vi "HFRR ADV v07 new software.vi"() -> ()   [LabVIEW 2025] (continued)
              n1803 = String Subset(string=w2037, offset (0)=85) -> (substring=w2039:string)  [unwired: 1 in]
              n1804 = String Subset(string=w2037, offset (0)=35, length (rest)=9 ("length (rest)")) -> (substring=w2060:string)
              n1805 = String Subset(string=w2037, offset (0)=55, length (rest)=9 ("length (rest)")) -> (substring=w2045:string)
              n1806 = String Subset(string=w2037, offset (0)=25) -> (substring=w2041:string)  [unwired: 1 in]
              n1807 = String Subset(string=w2037, offset (0)=15, length (rest)=9 ("length (rest)")) -> (substring=w2066:string)
              n1808 = String Subset(string=w2037, offset (0)=0, length (rest)=14 ("length (rest)")) -> (substring=w2063:string)
              n1809 = String Subset(string=w2037, offset (0)=45, length (rest)=9 ("length (rest)")) -> (substring=w2050:string)
              n1810 = String Subset(string=w2037, offset (0)=65, length (rest)=9 ("length (rest)")) -> (substring=w2056:string)
              n1811 = Fract/Exp String To Number(string=w2039) -> (number=w2036:dbl)  [unwired: 3 in, 1 out]
              n1812 = Fract/Exp String To Number(string=w2060) -> (number=w2058:dbl)  [unwired: 3 in, 1 out]
              n1813 = Fract/Exp String To Number(string=w2045) -> (number=w2043:dbl)  [unwired: 3 in, 1 out]
              n1814 = Fract/Exp String To Number(string=w2041) -> (number=w2040:dbl)  [unwired: 3 in, 1 out]
              n1815 = Fract/Exp String To Number(string=w2066) -> (number=w2057:dbl)  [unwired: 3 in, 1 out]
              n1816 = Fract/Exp String To Number(string=w2063) -> (number=w2059:dbl)  [unwired: 3 in, 1 out]
              n1817 = Fract/Exp String To Number(string=w2050) -> (number=w2047:dbl)  [unwired: 3 in, 1 out]
              n1818 = Fract/Exp String To Number(string=w2056) -> (number=w2053:dbl)  [unwired: 3 in, 1 out]
              n1819 = Add(x=w2053, y=0.0) -> (x+y=w2051:dbl)
            }
            n1820 = String To Path(string=w1896) -> (path=w1994:path)
            n1821 = String To Path(string=w1894) -> (path=w1988:path)
            n1822 = local read "Numeric 11"() -> (w1978:i32)
            n1823 = local read "Numeric 13"() -> (w1980:i32)
            n1824 = Open/Create/Replace File "Open File"(file path (use dialog)=w1994) -> (refnum out=w1992:refnum<file>, error out=w1991:errorcluster)  [unwired: 5 in, 1 out]
            n1825 = Open/Create/Replace File "Open File"(file path (use dialog)=w1988) -> (refnum out=w1987:refnum<file>, error out=w1986:errorcluster)  [unwired: 5 in, 1 out]
            n1826 = for {
              N: w1978 -> [_]
              tunnel: w1992 -> [w2107]
              tunnel: w1991 -> [w2106]
              tunnel: [w2096] -> w1958 mode=indexing
              tunnel: [w2094] -> w1956 mode=indexing
              tunnel: [w2095] -> w1951 mode=indexing
              tunnel: w1977 -> [_]
              tunnel: [w2088] -> w1953 mode=indexing
              tunnel: [w2084] -> w1929 mode=indexing
              tunnel: [w2080] -> w1904 mode=indexing
              tunnel: [w2076] -> w1885 mode=indexing
              tunnel: [w2071] -> w1843 mode=indexing
              (unwired) TRUE ("line mode (F)")
              n1827 = Read from Text File "Read File"(file (use dialog)=w2107, error in=w2106) -> (text=w2072:string)  [unwired: 2 in, 3 out]
              n1828 = local write "String 7"(w2072) -> ()
              n1829 = String Subset(string=w2072, offset (0)=85, length (rest)=9 ("length (rest)")) -> (substring=w2075:string)
              n1830 = String Subset(string=w2072, offset (0)=35, length (rest)=9 ("length (rest)")) -> (substring=w2097:string)
              n1831 = String Subset(string=w2072, offset (0)=55, length (rest)=9 ("length (rest)")) -> (substring=w2083:string)
              n1832 = String Subset(string=w2072, offset (0)=25, length (rest)=9 ("length (rest)")) -> (substring=w2077:string)
              n1833 = String Subset(string=w2072, offset (0)=45, length (rest)=9 ("length (rest)")) -> (substring=w2085:string)
              n1834 = String Subset(string=w2072, offset (0)=0, length (rest)=14 ("length (rest)")) -> (substring=w2100:string)
              n1835 = String Subset(string=w2072, offset (0)=15, length (rest)=9 ("length (rest)")) -> (substring=w2103:string)
              n1836 = String Subset(string=w2072, offset (0)=65, length (rest)=9 ("length (rest)")) -> (substring=w2089:string)
              n1837 = Fract/Exp String To Number(string=w2075) -> (number=w2071:dbl)  [unwired: 3 in, 1 out]
              n1838 = Fract/Exp String To Number(string=w2097) -> (number=w2095:dbl)  [unwired: 3 in, 1 out]
              n1839 = Fract/Exp String To Number(string=w2083) -> (number=w2080:dbl)  [unwired: 3 in, 1 out]
              n1840 = Fract/Exp String To Number(string=w2077) -> (number=w2076:dbl)  [unwired: 3 in, 1 out]
              n1841 = Fract/Exp String To Number(string=w2085) -> (number=w2084:dbl)  [unwired: 3 in, 1 out]
              n1842 = Fract/Exp String To Number(string=w2100) -> (number=w2096:dbl)  [unwired: 3 in, 1 out]
              n1843 = Fract/Exp String To Number(string=w2103) -> (number=w2094:dbl)  [unwired: 3 in, 1 out]
              n1844 = Fract/Exp String To Number(string=w2089) -> (number=w2092:dbl)  [unwired: 3 in, 1 out]
              n1845 = Add(x=w2092, y=0.0) -> (x+y=w2088:dbl)
            }
            n1846 = for {
              N: w1980 -> [_]
              tunnel: w1987 -> [w2035]
              tunnel: w1986 -> [w2034]
              tunnel: [w2024] -> w1940 mode=indexing
              tunnel: [w2023] -> w1933 mode=indexing
              tunnel: w1977 -> [_]
              tunnel: [w2012] -> w1938 mode=indexing
              tunnel: [w2017] -> w1935 mode=indexing
              tunnel: [w2013] -> w1925 mode=indexing
              tunnel: [w2008] -> w1900 mode=indexing
              tunnel: [w2004] -> w1881 mode=indexing
              tunnel: [w1999] -> w1841 mode=indexing
              (unwired) 1.0 ("x")
              (unwired) TRUE ("line mode (F)")
              n1847 = Read from Text File "Read File"(file (use dialog)=w2035, error in=w2034) -> (text=w2000:string)  [unwired: 2 in, 3 out]
              n1848 = local write "String 12"(w2000) -> ()
              n1849 = String Subset(string=w2000, offset (0)=85, length (rest)=9 ("length (rest)")) -> (substring=w2002:string)
              n1850 = String Subset(string=w2000, offset (0)=35, length (rest)=9 ("length (rest)")) -> (substring=w2025:string)
              n1851 = String Subset(string=w2000, offset (0)=55, length (rest)=9 ("length (rest)")) -> (substring=w2010:string)
              n1852 = String Subset(string=w2000, offset (0)=25, length (rest)=9 ("length (rest)")) -> (substring=w2006:string)
              n1853 = String Subset(string=w2000, offset (0)=45, length (rest)=9 ("length (rest)")) -> (substring=w2015:string)
              n1854 = String Subset(string=w2000, offset (0)=15, length (rest)=9 ("length (rest)")) -> (substring=w2031:string)
              n1855 = String Subset(string=w2000, offset (0)=0, length (rest)=14 ("length (rest)")) -> (substring=w2028:string)
              n1856 = String Subset(string=w2000, offset (0)=65, length (rest)=9 ("length (rest)")) -> (substring=w2018:string)
              n1857 = Fract/Exp String To Number(string=w2002) -> (number=w1999:dbl)  [unwired: 3 in, 1 out]
              n1858 = Fract/Exp String To Number(string=w2025) -> (number=w2023:dbl)  [unwired: 3 in, 1 out]
              n1859 = Fract/Exp String To Number(string=w2010) -> (number=w2008:dbl)  [unwired: 3 in, 1 out]
              n1860 = Fract/Exp String To Number(string=w2006) -> (number=w2004:dbl)  [unwired: 3 in, 1 out]
              n1861 = Fract/Exp String To Number(string=w2015) -> (number=w2013:dbl)  [unwired: 3 in, 1 out]
              n1862 = Fract/Exp String To Number(string=w2031) -> (number=w2012:dbl)  [unwired: 3 in, 1 out]
              n1863 = Fract/Exp String To Number(string=w2028) -> (number=w2024:dbl)  [unwired: 3 in, 1 out]
              n1864 = Fract/Exp String To Number(string=w2018) -> (number=w2021:dbl)  [unwired: 3 in, 1 out]
              n1865 = Add(x=w2021, y=0.0) -> (x+y=w2017:dbl)
            }
            n1866 = Delete From Array(array=w1883, index=0) -> (array with subset deleted=w1856:dbl[])  [unwired: 1 in, 1 out]
            n1867 = Delete From Array(array=w1946, index=0) -> (array with subset deleted=w1919:dbl[])  [unwired: 1 in, 1 out]
            n1868 = Delete From Array(array=w1926, index=0) -> (array with subset deleted=w1914:dbl[])  [unwired: 1 in, 1 out]
            n1869 = Delete From Array(array=w1944, index=0) -> (array with subset deleted=w1945:dbl[])  [unwired: 1 in, 1 out]
            n1870 = call-poly <vilib>:"Mean.vi"("X"=w1856) -> ("mean"=→"КОФ2 4":dbl)  [unwired: 1 out]
            n1871 = call-poly <vilib>:"Mean.vi"("X"=w1919) -> ("mean"=→"КОФ3":dbl)  [unwired: 1 out]
            n1872 = call-poly <vilib>:"Mean.vi"("X"=w1914) -> ("mean"=→"CP3":dbl)  [unwired: 1 out]
            n1873 = Delete From Array(array=w1908, index=0) -> (array with subset deleted=w1835:dbl[])  [unwired: 1 in, 1 out]
            n1874 = Delete From Array(array=w1847, index=0) -> (array with subset deleted=w1834:dbl[])  [unwired: 1 in, 1 out]
            n1875 = Delete From Array(array=w1887, index=0) -> (array with subset deleted=w1858:dbl[])  [unwired: 1 in, 1 out]
            n1876 = Delete From Array(array=w1965, index=0) -> (array with subset deleted=w1920:dbl[])  [unwired: 1 in, 1 out]
            n1877 = Delete From Array(array=w1931, index=0) -> (array with subset deleted=w1916:dbl[])  [unwired: 1 in, 1 out]
            "array w/ subset deleted" <- w1916
            n1878 = Delete From Array(array=w1962, index=0) -> (array with subset deleted=w1963:dbl[])  [unwired: 1 in, 1 out]
            n1879 = call-poly <vilib>:"Mean.vi"("X"=w1858) -> ("mean"=→"КОФ2 2":dbl)  [unwired: 1 out]
            n1880 = call-poly <vilib>:"Mean.vi"("X"=w1920) -> ("mean"=→"КОФ1":dbl)  [unwired: 1 out]
            n1881 = Bundle "Bundle"(w1835, w1834) -> (w1840:cluster{dbl[], dbl[]})  [unwired: 1 in]
            n1882 = Bundle "Bundle"(w1835, w1963) -> (w1827:cluster{dbl[], dbl[]})  [unwired: 1 in]
            n1883 = Delete From Array(array=w1842, index=0) -> (array with subset deleted=w1830:dbl[])  [unwired: 1 in, 1 out]
            n1884 = Delete From Array(array=w1843, index=0) -> (array with subset deleted=w1832:dbl[])  [unwired: 1 in, 1 out]
            n1885 = Delete From Array(array=w1953, index=0) -> (array with subset deleted=w1954:dbl[])  [unwired: 1 in, 1 out]
            n1886 = Delete From Array(array=w1841, index=0) -> (array with subset deleted=w1828:dbl[])  [unwired: 1 in, 1 out]
            n1887 = Delete From Array(array=w1935, index=0) -> (array with subset deleted=w1936:dbl[])  [unwired: 1 in, 1 out]
            n1888 = Delete From Array(array=w1960, index=0) -> (array with subset deleted=w1866:dbl[])  [unwired: 1 in, 1 out]
            n1889 = Delete From Array(array=w1906, index=0) -> (array with subset deleted=w1862:dbl[])  [unwired: 1 in, 1 out]
            n1890 = Delete From Array(array=w1942, index=0) -> (array with subset deleted=w1864:dbl[])  [unwired: 1 in, 1 out]
            n1891 = Delete From Array(array=w1902, index=0) -> (array with subset deleted=w1860:dbl[])  [unwired: 1 in, 1 out]
            n1892 = Delete From Array(array=w1951, index=0) -> (array with subset deleted=w1865:dbl[])  [unwired: 1 in, 1 out]
            n1893 = Delete From Array(array=w1904, index=0) -> (array with subset deleted=w1861:dbl[])  [unwired: 1 in, 1 out]
            n1894 = Delete From Array(array=w1885, index=0) -> (array with subset deleted=w1857:dbl[])  [unwired: 1 in, 1 out]
            n1895 = Delete From Array(array=w1929, index=0) -> (array with subset deleted=w1915:dbl[])  [unwired: 1 in, 1 out]
            n1896 = Delete From Array(array=w1956, index=0) -> (array with subset deleted=w1917:dbl[])  [unwired: 1 in, 1 out]
            n1897 = Delete From Array(array=w1933, index=0) -> (array with subset deleted=w1863:dbl[])  [unwired: 1 in, 1 out]
            n1898 = Delete From Array(array=w1900, index=0) -> (array with subset deleted=w1859:dbl[])  [unwired: 1 in, 1 out]
            n1899 = Delete From Array(array=w1881, index=0) -> (array with subset deleted=w1855:dbl[])  [unwired: 1 in, 1 out]
            n1900 = Delete From Array(array=w1925, index=0) -> (array with subset deleted=w1913:dbl[])  [unwired: 1 in, 1 out]
            n1901 = Delete From Array(array=w1938, index=0) -> (array with subset deleted=w1918:dbl[])  [unwired: 1 in, 1 out]
            n1902 = Delete From Array(array=w1948, index=0) -> (array with subset deleted=w1831:dbl[])  [unwired: 1 in, 1 out]
            n1903 = Delete From Array(array=w1958, index=0) -> (array with subset deleted=w1833:dbl[])  [unwired: 1 in, 1 out]
            n1904 = Delete From Array(array=w1940, index=0) -> (array with subset deleted=w1829:dbl[])  [unwired: 1 in, 1 out]
            n1905 = Bundle "Bundle"(w1835, w1866) -> (w1853:cluster{dbl[], dbl[]})  [unwired: 1 in]
            n1906 = Bundle "Bundle"(w1835, w1920) -> (w1854:cluster{dbl[], dbl[]})  [unwired: 1 in]
            n1907 = Bundle "Bundle"(w1866, w1862) -> (w1868:cluster{dbl[], dbl[]})  [unwired: 1 in]
            n1908 = Bundle "Bundle"(w1831, w1830) -> (w1838:cluster{dbl[], dbl[]})  [unwired: 1 in]
            n1909 = Bundle "Bundle"(w1864, w1860) -> (w1870:cluster{dbl[], dbl[]})  [unwired: 1 in]
            n1910 = Bundle "Bundle"(w1831, w1864) -> (w1974:cluster{dbl[], dbl[]})  [unwired: 1 in]
            n1911 = Bundle "Bundle"(w1831, w1860) -> (w1898:cluster{dbl[], dbl[]})  [unwired: 1 in]
            n1912 = Bundle "Bundle"(w1831, w1919) -> (w1984:cluster{dbl[], dbl[]})  [unwired: 1 in]
            n1913 = Bundle "Bundle"(w1831, w1914) -> (w1922:cluster{dbl[], dbl[]})  [unwired: 1 in]
            n1914 = Bundle "Bundle"(w1831, w1945) -> (w1969:cluster{dbl[], dbl[]})  [unwired: 1 in]
            n1915 = Bundle "Bundle"(w1865, w1861) -> (w1869:cluster{dbl[], dbl[]})  [unwired: 1 in]
            n1916 = Bundle "Bundle"(w1833, w1832) -> (w1839:cluster{dbl[], dbl[]})  [unwired: 1 in]
            n1917 = Bundle "Bundle"(w1833, w1865) -> (w1976:cluster{dbl[], dbl[]})  [unwired: 1 in]
            n1918 = Bundle "Bundle"(w1833, w1861) -> (w1899:cluster{dbl[], dbl[]})  [unwired: 1 in]
            n1919 = Bundle "Bundle"(w1833, w1915) -> (w1923:cluster{dbl[], dbl[]})  [unwired: 1 in]
            n1920 = Bundle "Bundle"(w1833, w1917) -> (w1985:cluster{dbl[], dbl[]})  [unwired: 1 in]
            n1921 = Bundle "Bundle"(w1833, w1954) -> (w1967:cluster{dbl[], dbl[]})  [unwired: 1 in]
            n1922 = Bundle "Bundle"(w1863, w1859) -> (w1871:cluster{dbl[], dbl[]})  [unwired: 1 in]
            n1923 = Bundle "Bundle"(w1829, w1828) -> (w1837:cluster{dbl[], dbl[]})  [unwired: 1 in]
            n1924 = Bundle "Bundle"(w1829, w1863) -> (w1975:cluster{dbl[], dbl[]})  [unwired: 1 in]
            n1925 = Bundle "Bundle"(w1829, w1859) -> (w1897:cluster{dbl[], dbl[]})  [unwired: 1 in]
            n1926 = Bundle "Bundle"(w1829, w1913) -> (w1921:cluster{dbl[], dbl[]})  [unwired: 1 in]
            n1927 = Bundle "Bundle"(w1829, w1918) -> (w1983:cluster{dbl[], dbl[]})  [unwired: 1 in]
            n1928 = Bundle "Bundle"(w1829, w1936) -> (w1968:cluster{dbl[], dbl[]})  [unwired: 1 in]
            n1929 = call-poly <vilib>:"Mean.vi"("X"=w1916) -> ("mean"=→"CP1":dbl)  [unwired: 1 out]
            n1930 = call-poly <vilib>:"Mean.vi"("X"=w1857) -> ("mean"=→"КОФ2 3":dbl)  [unwired: 1 out]
            n1931 = call-poly <vilib>:"Mean.vi"("X"=w1915) -> ("mean"=→"CP2":dbl)  [unwired: 1 out]
            n1932 = call-poly <vilib>:"Mean.vi"("X"=w1917) -> ("mean"=→"КОФ2":dbl)  [unwired: 1 out]
            n1933 = call-poly <vilib>:"Mean.vi"("X"=w1855) -> ("mean"=→"КОФ2 5":dbl)  [unwired: 1 out]
            n1934 = call-poly <vilib>:"Mean.vi"("X"=w1913) -> ("mean"=→"CP4":dbl)  [unwired: 1 out]
            n1935 = call-poly <vilib>:"Mean.vi"("X"=w1918) -> ("mean"=→"КОФ4":dbl)  [unwired: 1 out]
            n1936 = Bundle "Bundle"(w1835, w1862) -> (w1826:cluster{dbl[], dbl[]})  [unwired: 1 in]
            n1937 = Bundle "Bundle"(w1835, w1916) -> (w1849:cluster{dbl[], dbl[]})  [unwired: 1 in]
            n1938 = Build Array "Build Array"(w1826, w1849) -> (w1852:cluster{dbl[], dbl[]}[])
            "XY Graph 17" <- w1852
            n1939 = Build Array "Build Array"(w1840, w1839, w1838, w1837) -> (→"Frequency ( Hz )":cluster{dbl[], dbl[]}[])
            n1940 = Build Array "Build Array"(w1868, w1869, w1870, w1871) -> (→"Air Temp ( °C ) vs Humidity ( % RH )":cluster{dbl[], dbl[]}[])
            n1941 = Build Array "Build Array"(w1853, w1976, w1974, w1975) -> (→"Air Temperature  ( °C )":cluster{dbl[], dbl[]}[])
            n1942 = Build Array "Build Array"(w1826, w1899, w1898, w1897) -> (→"Humidity ( %RH )":cluster{dbl[], dbl[]}[])
            n1943 = Build Array "Build Array"(w1854, w1985, w1984, w1983) -> (→"Coefficient Of Friction":cluster{dbl[], dbl[]}[])
            n1944 = Build Array "Build Array"(w1849, w1923, w1922, w1921) -> (→"Sample Temperature ( °C )":cluster{dbl[], dbl[]}[])
            n1945 = Build Array "Build Array"(w1827, w1967, w1969, w1968) -> (→"XY Graph 13":cluster{dbl[], dbl[]}[])
            n1946 = Bundle "Bundle"(w1835, w1858) -> (w1880:cluster{dbl[], dbl[]})  [unwired: 1 in]
            n1947 = Bundle "Bundle"(w1831, w1856) -> (w1878:cluster{dbl[], dbl[]})  [unwired: 1 in]
            n1948 = Bundle "Bundle"(w1833, w1857) -> (w1879:cluster{dbl[], dbl[]})  [unwired: 1 in]
            n1949 = Bundle "Bundle"(w1829, w1855) -> (w1877:cluster{dbl[], dbl[]})  [unwired: 1 in]
            n1950 = Build Array "Build Array"(w1880, w1879, w1878, w1877) -> (→"Stroke ( mm )":cluster{dbl[], dbl[]}[])
            n1951 = local write "XY Graph 16"(w1852) -> ()
          }
          frame #2 {
          }
          frame #3 {
            n1952 = local write "Numeric 8"(0 ("Numeric 8")) -> ()
            n1953 = local write "Numeric 11"(0 ("Numeric 11")) -> ()
            n1954 = local write "Numeric 12"(0 ("Numeric 12")) -> ()
            n1955 = local write "Numeric 13"(0 ("Numeric 13")) -> ()
            n1956 = property on="OPEN" class="Bool (strict)"("Visible"=TRUE) -> ()  [unwired: 2 in, 2 out]
            n1957 = local read "String Control 2"() -> (w2152:string)
            n1958 = local read "String Control 4"() -> (w2151:string)
            n1959 = local read "String Control 6"() -> (w2150:string)
            n1960 = local read "String Control 8"() -> (w2149:string)
            n1961 = Match Pattern(string=w2152, regular expression="Samples / cycle :- ") -> (after substring=w2166:string)  [unwired: 1 in, 3 out]
            n1962 = Match Pattern(string=w2152, regular expression="Frequency :- ") -> (after substring=w2185:string)  [unwired: 1 in, 3 out]
            n1963 = Match Pattern(string=w2151, regular expression="Samples / cycle :- ") -> (after substring=w2162:string)  [unwired: 1 in, 3 out]
            n1964 = Match Pattern(string=w2151, regular expression="Frequency :- ") -> (after substring=w2180:string)  [unwired: 1 in, 3 out]
            n1965 = Match Pattern(string=w2150, regular expression="Samples / cycle :- ") -> (after substring=w2158:string)  [unwired: 1 in, 3 out]
            n1966 = Match Pattern(string=w2150, regular expression="Frequency :- ") -> (after substring=w2175:string)  [unwired: 1 in, 3 out]
            n1967 = Match Pattern(string=w2149, regular expression="Samples / cycle :- ") -> (after substring=w2154:string)  [unwired: 1 in, 3 out]
            n1968 = Match Pattern(string=w2149, regular expression="Frequency :- ") -> (after substring=w2170:string)  [unwired: 1 in, 3 out]
            n1969 = String Subset(string=w2166, length (rest)=6 ("length (rest)")) -> (substring=w2168:string)  [unwired: 1 in]
            n1970 = String Subset(string=w2185, length (rest)=9 ("length (rest)")) -> (substring=w2187:string)  [unwired: 1 in]
            n1971 = String Subset(string=w2162, length (rest)=6 ("length (rest)")) -> (substring=w2164:string)  [unwired: 1 in]
            n1972 = String Subset(string=w2180, length (rest)=9 ("length (rest)")) -> (substring=w2182:string)  [unwired: 1 in]
            n1973 = String Subset(string=w2158, length (rest)=6 ("length (rest)")) -> (substring=w2160:string)  [unwired: 1 in]
            n1974 = String Subset(string=w2175, length (rest)=9 ("length (rest)")) -> (substring=w2177:string)  [unwired: 1 in]
            n1975 = String Subset(string=w2154, length (rest)=6 ("length (rest)")) -> (substring=w2156:string)  [unwired: 1 in]
            n1976 = String Subset(string=w2170, length (rest)=9 ("length (rest)")) -> (substring=w2172:string)  [unwired: 1 in]
            n1977 = Fract/Exp String To Number(string=w2168) -> (number=w2148:dbl)  [unwired: 3 in, 1 out]
            n1978 = Fract/Exp String To Number(string=w2187) -> (number=w2188:dbl)  [unwired: 3 in, 1 out]
            n1979 = Fract/Exp String To Number(string=w2164) -> (number=w2147:dbl)  [unwired: 3 in, 1 out]
            n1980 = Fract/Exp String To Number(string=w2182) -> (number=w2183:dbl)  [unwired: 3 in, 1 out]
            n1981 = Fract/Exp String To Number(string=w2160) -> (number=w2146:dbl)  [unwired: 3 in, 1 out]
            n1982 = Fract/Exp String To Number(string=w2177) -> (number=w2178:dbl)  [unwired: 3 in, 1 out]
            n1983 = Fract/Exp String To Number(string=w2156) -> (number=w2145:dbl)  [unwired: 3 in, 1 out]
            n1984 = Fract/Exp String To Number(string=w2172) -> (number=w2173:dbl)  [unwired: 3 in, 1 out]
            n1985 = local write "sample1"(w2148) -> ()
            n1986 = local write "freq1"(w2188) -> ()
            n1987 = local write "sample2"(w2147) -> ()
            n1988 = local write "freq2"(w2183) -> ()
            n1989 = local write "sample3"(w2146) -> ()
            n1990 = local write "freq3"(w2178) -> ()
            n1991 = local write "sample4"(w2145) -> ()
            n1992 = local write "freq 4"(w2173) -> ()
          }
        }
      }
    }
    n1993 = case shown="True" w1637 {
      selector: w1637 -> [_ w1765]
      frame False {
      }
      frame True {
        n1994 = Not(x=w1765) -> (.not. x?=w1761:bool)
        n1995 = local write "service 3"(w1761) -> ()
        n1996 = local write "OPEN 6"(w1761) -> ()
        n1997 = call <vilib>:"System Exec.vi"("wait until completion? (T)"=TRUE, "command line"="C:\\LAB-IQ\\Scar View.exe") -> ("error out"=→"error out 5":errorcluster)  [unwired: 6 in, 3 out]
      }
    }
    n1998 = case shown="\"Acquire\", Default" w1648 {
      frame "Acquire", Default {
        w2661 = 0.2 ("y")
        w2666 = 1.0 ("y")
        w2667 = 0.8 ("y")
        # "Elapsed time\ncof\nstroke\nAir temp\nTemp\nHumidity"
        n1999 = disable-structure shown="Disabled" {
          frame Disabled {
            n2000 = local read "Flag"() -> (w2684:dbl)
            n2001 = local read "RUN"() -> (w2681:bool)
            n2002 = Not(x=w2681) -> (.not. x?=w2680:bool)
            n2003 = Equal?(x=w2684, y=10.0) -> (x = y?=w2682:bool)
            n2004 = And(x=w2682, y=w2680) -> (x .and. y?=w2679:bool)
            n2005 = case shown="True" w2679 {
              frame False {
              }
              frame True {
                w2685 = FALSE ("Heater Button")
                n2006 = local write "Humidity"(w2685) -> ()
                n2007 = local write "Heater Button"(w2685) -> ()
              }
            }
          }
          frame Enabled {
          }
        }
        n2008 = disable-structure shown="Disabled" {
          frame Disabled {
            n2009 = case shown="True" {
              selector: _ -> [_ _]
              frame False {
              }
              frame True {
                w2776 = TRUE ("Heater")
                n2010 = local write "Humidity"(w2776) -> ()
                n2011 = local write "Heater Button"(w2776) -> ()
                n2012 = local read "TEST STANDARD"() -> (w2779:T3)
                n2013 = local read "TEST STANDARD"() -> (w2774:T3)
                n2014 = Equal?(x=w2779, y=enum16{"ASTM D6079", "ISO 12156", "Custom"}."ISO 12156" ("Test Standard")) -> (x = y?=w2777:bool)
                n2015 = Equal?(x=w2774, y=enum16{"ASTM D6079", "ISO 12156", "Custom"}."ASTM D6079" ("Test Standard")) -> (x = y?=w2773:bool)
                n2016 = case shown="True" w2777 {
                  frame False {
                  }
                  frame True {
                    n2017 = local write "Heater"(TRUE ("Heater")) -> ()
                    n2018 = local write "airtempflg"(FALSE ("airtempflg")) -> ()
                  }
                }
                n2019 = case shown="True" w2773 {
                  frame False {
                  }
                  frame True {
                    n2020 = local write "Heater"(FALSE ("Heater")) -> ()
                    n2021 = local write "airtempflg"(TRUE ("airtempflg")) -> ()
                  }
                }
              }
            }
          }
          frame Enabled {
          }
        }
        n2022 = stacked-sequence {
          frame #0 {
            n2023 = case shown="True" "RST FF" {
              frame False {
              }
              frame True {
                w2842 = 0.0 ("X Scale.Range:Maximum")
                n2024 = property on="Frictional Force ( N )" class="WFChart (strict)"("XScale.Maximum"=600.0 ("X Scale.Range:Maximum"), "XScale.Minimum"=w2842, "YScale.Maximum"=10.0 ("Y Scale.Range:Maximum"), "YScale.Minimum"=w2842) -> ()  [unwired: 2 in, 2 out]
              }
            }
          }
          frame #1 {
            n2025 = case shown="True" "RST TEMP" {
              frame False {
              }
              frame True {
                n2026 = property on="Temperature ( Deg C )" class="WFChart (strict)"("XScale.Minimum"=0.0 ("X Scale.Range:Minimum"), "XScale.Maximum"=600.0 ("X Scale.Range:Maximum"), "YScale.Minimum"=0.0 ("Y Scale.Range:Minimum"), "YScale.Maximum"=100.0 ("Y Scale.Range:Maximum")) -> ()  [unwired: 2 in, 2 out]
              }
            }
          }
          frame #2 {
            n2027 = case shown="True" "RSTCOF" {
              frame False {
              }
              frame True {
                n2028 = property on="Coefficient of Friction" class="WFChart (strict)"("XScale.Minimum"=0.0 ("X Scale.Range:Minimum"), "XScale.Maximum"=600.0 ("X Scale.Range:Maximum"), "YScale.Maximum"=1.0 ("X Scale.Range:Minimum"), "YScale.Minimum"=0.0 ("X Scale.Range:Minimum")) -> ()  [unwired: 2 in, 2 out]
              }
            }
          }
          frame #3 {
            n2029 = case shown="True" "RSTCOF 2" {
              frame False {
              }
              frame True {
                (unwired) 100.0 ("Y Scale.Range:Maximum")
                (unwired) 0.0 ("Y Scale.Range:Minimum")
                (unwired) 600.0 ("X Scale.Range:Maximum")
                (unwired) 0.0 ("X Scale.Range:Minimum")
              }
            }
          }
          frame #4 {
            n2030 = case shown="True" "RSTCOF 3" {
              frame False {
              }
              frame True {
                n2031 = property on="Electrical Contact Resistance ( % )" class="WFChart (strict)"("XScale.Minimum"=0.0 ("X Scale.Range:Minimum"), "XScale.Maximum"=600.0 ("X Scale.Range:Maximum"), "YScale.Minimum"=0.0 ("Y Scale.Range:Minimum"), "YScale.Maximum"=100.0 ("Y Scale.Range:Maximum")) -> ()  [unwired: 2 in, 2 out]
              }
            }
          }
        }
        n2032 = disable-structure shown="Disabled" {
          frame Disabled {
            n2033 = case shown="True" {
              selector: _ -> [_ _]
              frame False {
              }
              frame True {
                n2034 = local read "zflag 2"() -> (w2743:dbl)
                n2035 = local read "yflag"() -> (w2745:dbl)
                n2036 = Equal?(x=w2745, y=2.0 ("tflag")) -> (x = y?=w2747:bool)
                n2037 = Equal?(x=w2743, y=3.0 ("tflag")) -> (x = y?=w2746:bool)
                n2038 = And(x=w2747, y=w2746) -> (x .and. y?=w2741:bool)
                n2039 = case shown="True" w2741 {
                  frame False {
                  }
                  frame True {
                    w2772 = 0.0 ("zflag")
                    n2040 = local write "zflag"(w2772) -> ()
                    n2041 = local write "zflag 2"(w2772) -> ()
                    n2042 = Delete(path (use dialog)=path "C:/LAB-IQ-NXT/WO 2449 TT.sig" ("file path (dialog if empty)")) -> (deleted path=w2771:path)  [unwired: 4 in, 2 out]
                    n2043 = Delete(path (use dialog)=path "C:/LAB-IQ-NXT/WO 2449 TRH.sig" ("file path (dialog if empty)")) -> (deleted path=w2766:path)  [unwired: 4 in, 2 out]
                    n2044 = local read "SEN.RUN HRS"() -> (w2758:dbl)
                    n2045 = local read "SENSOR TIME"() -> (w2756:dbl)
                    n2046 = call <vilib>:"compatOverwrite.vi"("overwrite (F)"=TRUE) -> ("overwrite?"=w2748:T27)
                    n2047 = call <vilib>:"compatOverwrite.vi"("overwrite (F)"=TRUE) -> ("overwrite?"=w2752:T27)
                    n2048 = local read "Total No. of Tests"() -> (w2759:dbl)
                    n2049 = Add(x=w2756, y=w2758) -> (x+y=w2757:dbl)
                    "SEN.RUN HRS" <- w2757
                    n2050 = Open/Create/Replace File(file path (use dialog)=w2771, operation (0:open)=w2748) -> (refnum out=w2749:refnum<file>, error out=w2750:errorcluster)  [unwired: 4 in, 1 out]
                    n2051 = Open/Create/Replace File(file path (use dialog)=w2766, operation (0:open)=w2752) -> (refnum out=w2753:refnum<file>, error out=w2754:errorcluster)  [unwired: 4 in, 1 out]
                    n2052 = Deny Access(4:w2750, 6:T25."deny none" ("deny mode (2)"), 7:w2749) -> (3:w2770:refnum<file>)  [unwired: 1 out]
                    n2053 = Deny Access(4:w2754, 6:T25."deny none" ("deny mode (2)"), 7:w2753) -> (3:w2762:refnum<file>)  [unwired: 1 out]
                    n2054 = Number To Decimal String(number=w2759) -> (decimal integer string=w2767:string)  [unwired: 1 in]
                    n2055 = Number To Decimal String(number=w2757) -> (decimal integer string=w2763:string)  [unwired: 1 in]
                    n2056 = Write to Binary File(file (use dialog)=w2770, data=w2767, 5:FALSE ("prepend array or string size? (T)")) -> ()  [unwired: 3 in, 3 out]
                    n2057 = Write to Binary File(file (use dialog)=w2762, data=w2763, 5:FALSE ("prepend array or string size? (T)")) -> ()  [unwired: 3 in, 3 out]
                  }
                }
              }
            }
          }
          frame Enabled {
          }
        }
        n2058 = local read "RUN"() -> (w2670:bool)
        n2059 = local read "run replace"() -> (w2674:bool)
        n2060 = local read "run replace"() -> (w2673:bool)
        n2061 = case shown="True" w2670 {
          frame False {
            n2062 = local write "run replace"(FALSE ("run replace")) -> ()
          }
          frame True {
            "run replace" <- TRUE ("run replace")
          }
        }
        n2063 = local read "RUN"() -> (w2678:bool)
        n2064 = local read "Set Temp"() -> (w2640:dbl)
        n2065 = local read "SetTemp"() -> (w2642:dbl)
        n2066 = case shown="False" w2678 {
          tunnel: [FALSE ("TEST RUNNING") TRUE ("TEST RUNNING")] -> w2677
          frame False {
            w2861 = 0.0 ("Flag")
            n2067 = local write "Elapsed time"(0.0 ("elapsedtime")) -> ()
            n2068 = local write "Time Remaining"(w2861) -> ()
            n2069 = local write "Flag"(w2861) -> ()
            n2070 = local write "Remaining Time"(w2861) -> ()
          }
          frame True {
            n2071 = local write "Flag"(10.0 ("Flag")) -> ()
          }
        }
        n2072 = case shown="False" w2674 {
          frame False {
            n2073 = local read "zflag"() -> (→"zflag 2":dbl)
            n2074 = local write "yflag"(2.0 ("tflag")) -> ()
            n2075 = local write "FLAG 4"(0.0 ("FLAG")) -> ()
          }
          frame True {
            n2076 = local write "yflag"(1.0 ("tflag")) -> ()
            n2077 = local write "zflag"(3.0 ("zflag")) -> ()
          }
        }
        n2078 = local read "acq 2"() -> (w2672:bool)
        n2079 = local read "AIR TEMP"() -> (w2635:dbl)
        n2080 = local read "Amb temp"() -> (w2639:dbl)
        n2081 = case shown="True" "Save & Continue" {
          frame False {
          }
          frame True {
            "acq 2" <- TRUE ("acq 2")
          }
        }
        n2082 = local read "Set Rh"() -> (w2641:dbl)
        n2083 = Add(x=w2642, y=w2667) -> (x+y=w2668:dbl)
        n2084 = Subtract(x=w2642, y=w2667) -> (x-y=w2669:dbl)
        n2085 = Add(x=w2640, y=w2661) -> (x+y=w2662:dbl)
        n2086 = Subtract(x=w2640, y=w2661) -> (x-y=w2663:dbl)
        n2087 = And(x=w2672, y=w2673) -> (x .and. y?=w2671:bool)
        n2088 = Greater Or Equal?(x=w2635, y=15.0) -> (x >= y?=w2636:bool)
        "powstat" <- w2636
        n2089 = local read "Humidity ( %RH )"() -> (w2638:dbl)
        n2090 = case shown="True" "Save & Continue" {
          frame False {
          }
          frame True {
            n2091 = while {
              tunnel: "0123456789abcdefghijklmnopqrstuvwxyzABCDEFGHIJKLMNOPQRSTUVWXYZ" ("string 2") -> [w2832]
              shift-right: [w2830] -> w2825
              shift-left: "" -> [w2829]
              i -> [w2839]
              stop <- w2838 stop-if-true
              n2092 = Random Number (0-1)() -> (number: 0 to 1=w2833:dbl)
              n2093 = Multiply(x=w2833, y=62.0) -> (x*y=w2835:dbl)
              n2094 = Decrement(x="Length") -> (x-1=w2828:i16)
              n2095 = To Word Integer(number=w2835) -> (16bit integer=w2836:i16)
              n2096 = String Subset(string=w2832, offset (0)=w2836, length (rest)=1 ("length (rest)")) -> (substring=w2831:string)
              n2097 = Greater Or Equal?(x=w2839, y=w2828) -> (x >= y?=w2838:bool)
              n2098 = Concatenate Strings(w2831, w2829) -> (w2830:string)
            }
            n2099 = local write "UUID"(w2825) -> ()
          }
        }
        n2100 = In Range and Coerce(upper limit=w2668, x=w2639, lower limit=w2669) -> (In Range?=w2658:bool)  [unwired: 1 out]
        n2101 = Add(x=w2641, y=w2666) -> (x+y=w2665:dbl)
        n2102 = Subtract(x=w2641, y=w2666) -> (x-y=w2664:dbl)
        n2103 = local read "TEMP"() -> (w2637:dbl)
        n2104 = case shown="True" "Save & Continue" {
          frame False {
          }
          frame True {
            n2105 = local read "Operator ID"() -> (w3149:string)
            n2106 = local read "FILE"() -> (w3155:string)
            n2107 = String Length(string=w3155) -> (length=w3153:i32)
            n2108 = String Length(string=w3149) -> (length=w3150:i32)
            n2109 = Greater?(x=w3153, y=0) -> (0:w3152:bool)
            n2110 = Greater?(x=w3150, y=0) -> (0:w3148:bool)
            n2111 = And(x=w3152, y=w3148) -> (x .and. y?=w3147:bool)
            n2112 = case shown="True" w3147 {
              frame False {
                n2113 = stacked-sequence {
                  frame #0 {
                    n2114 = One Button Dialog(message="Please Enter a File Name and Operator ID to save data !", button name ("OK")="Ok") -> ()  [unwired: 1 out]
                  }
                  frame #1 {
                    n2115 = local write "Save & Continue"(FALSE ("OK Button")) -> ()
                  }
                }
                n2116 = local write "Save & Continue"(FALSE ("OK Button")) -> ()
              }
              frame True {
                n2117 = stacked-sequence {
                  frame #0 {
                    n2118 = local read "FILE"() -> (w3161:string)
                    n2119 = call "file check.vi"("file name in"=w3161) -> ("file name out"=w3160:string)  [unwired: 9 in, 1 out]
                    n2120 = call <vilib>:"Application Directory.vi"() -> ("Application Directory"=w3171:path)
                    n2121 = Build Path(base path=w3171, name or relative path="data") -> (appended path=w3170:path)
                    n2122 = call <vilib>:"Trim Whitespace.vi"("string"=w3160) -> ("trimmed string"=w3168:string)  [unwired: 1 in]
                    n2123 = call <vilib>:"Trim Whitespace.vi"("string"=w3160) -> ("trimmed string"=w3169:string)  [unwired: 1 in]
                    n2124 = List Folder(path=w3170) -> (folder names=w3166:string[])  [unwired: 3 in, 3 out]
                    n2125 = Match Pattern(string=w3168, regular expression="_(") -> (before substring=w3165:string)  [unwired: 1 in, 3 out]
                    n2126 = for {
                      tunnel: w3166 -> [w3180] mode=indexing
                      tunnel: w3165 -> [w3178]
                      shift-right: [w3176] -> w3163
                      shift-left: bool[] [] -> [w3177]
                      n2127 = Match Pattern(string=w3180, regular expression="_(") -> (before substring=w3179:string)  [unwired: 1 in, 3 out]
                      n2128 = Equal?(x=w3179, y=w3178) -> (x = y?=w3175:bool)
                      n2129 = case shown="True" w3175 {
                        tunnel: w3175 -> [_ w3183]
                        tunnel: w3177 -> [w3182 w3185]
                        tunnel: [w3182 w3184] -> w3176
                        frame False {
                        }
                        frame True {
                          n2130 = Insert Into Array(array=w3185, new element=w3183) -> (w3184:bool[])  [unwired: 1 in]
                        }
                      }
                    }
                    n2131 = Equal?(x=w3166, y=w3165) -> (x = y?=w3174:bool[])
                    n2132 = Or Array Elements(Boolean array=w3174) -> (logical OR=w3173:bool)
                    n2133 = Array Size(array=w3163) -> (size(s)=w3162:i32)
                    n2134 = case shown="True" w3173 {
                      tunnel: w3169 -> [_ w3193]
                      tunnel: w3162 -> [_ w3186]
                      frame False {
                      }
                      frame True {
                        n2135 = Number To Decimal String(number=w3186) -> (decimal integer string=w3189:string)  [unwired: 1 in]
                        n2136 = Search/Split String(string=w3193, search string/char (-)="_(" ("regular expression")) -> (substring before match=w3191:string)  [unwired: 1 in, 2 out]
                        n2137 = Concatenate Strings(w3191, "_(" ("regular expression"), w3189, ")" ("regular expression")) -> (w3187:string)
                        n2138 = local write "FILE"(w3187) -> ()
                      }
                    }
                  }
                  frame #1 {
                    w3195 = 0.0
                    w3208 = cluster{"y":dbl, dbl, "y":dbl}[] [] ("History Data")
                    w3209 = FALSE ("Heater Button")
                    (unwired) ")!" ("string")
                    (unwired) ")" ("string")
                    w3207 = dbl[] [] ("History Data")
                    w3213 = "\r"
                    # "C:\\WinDucom\\Data\\"
                    # "C:\\LAB-IQ-NXT\\data"
                    n2139 = local write "Humidity ( %RH )"(w3195) -> ()
                    n2140 = local write "Frequency ( Hz )"(w3195) -> ()
                    n2141 = local write "Stroke 3"(w3195) -> ()
                    n2142 = local write "speedop"(0.0 ("PIDclk 2")) -> ()
                    n2143 = local write "Set Temp 2"(65.0 ("Set Temp 2")) -> ()
                    n2144 = local write "AIR TEMP"(w3195) -> ()
                    n2145 = local write "clk"(0.0 ("clk")) -> ()
                    n2146 = local write "Stroke 4"(w3195) -> ()
                    n2147 = local write "COF 2"(w3195) -> ()
                    n2148 = local write "TEMP"(w3195) -> ()
                    n2149 = local write "ecr 3"(w3195) -> ()
                    n2150 = local write "FF 3"(w3195) -> ()
                    n2151 = local write "FF 2"(w3195) -> ()
                    n2152 = property on="Humidity ( %RH )" class="WFChart (strict)"("History Data"=w3207) -> ()  [unwired: 2 in, 2 out]
                    n2153 = property on="Coefficient of Friction" class="WFChart (strict)"("History Data"=w3207) -> ()  [unwired: 2 in, 2 out]
                    n2154 = property on="Coefficient of Friction" class="WFChart (strict)"("History Data"=w3207) -> ()  [unwired: 2 in, 2 out]
                    n2155 = property on="Frictional Force ( N )" class="WFChart (strict)"("History Data"=w3207) -> ()  [unwired: 2 in, 2 out]
                    n2156 = property on="Electrical Contact Resistance ( % )" class="WFChart (strict)"("History Data"=w3207) -> ()  [unwired: 2 in, 2 out]
                    n2157 = property on="Electrical Contact Resistance ( % )" class="WFChart (strict)"("History Data"=w3207) -> ()  [unwired: 2 in, 2 out]
                    n2158 = property on="Temperature ( Deg C )" class="WFChart (strict)"("History Data"=w3207) -> ()  [unwired: 2 in, 2 out]
                    n2159 = property on="Frictional Force ( N )" class="WFChart (strict)"("History Data"=w3207) -> ()  [unwired: 2 in, 2 out]
                    n2160 = property on="Coefficient of Friction" class="WFChart (strict)"("History Data"=w3207) -> ()  [unwired: 2 in, 2 out]
                    n2161 = property on="Frictional Force ( N )" class="WFChart (strict)"("History Data"=w3207) -> ()  [unwired: 2 in, 2 out]
                    n2162 = property on="Electrical Contact Resistance ( % )" class="WFChart (strict)"("History Data"=w3207) -> ()  [unwired: 2 in, 2 out]
                    n2163 = property on="Temperature ( Deg C )" class="WFChart (strict)"("History Data"=w3207) -> ()  [unwired: 2 in, 2 out]
                    n2164 = property on="Humidity ( %RH )" class="WFChart (strict)"("History Data"=w3207) -> ()  [unwired: 2 in, 2 out]
                    n2165 = property on="Stroke ( mm )" class="WFChart (strict)"("History Data"=w3208) -> ()  [unwired: 2 in, 2 out]
                    n2166 = property on="Stroke ( mm )" class="WFChart (strict)"("History Data"=w3208) -> ()  [unwired: 2 in, 2 out]
                    n2167 = local write "Humidity"(w3209) -> ()
                    n2168 = local write "Heater Button"(w3209) -> ()
                    n2169 = local read "FILE"() -> (w3203:string)
                    n2170 = disable-structure shown="Enabled" {
                      disable-tunnel: [w3248 _] -> w3194
                      frame Enabled {
                        n2171 = local read "NORMAL LOAD"() -> (w3248:dbl)
                      }
                      frame Disabled {
                      }
                    }
                    n2172 = call "file check.vi"("file name in"=w3203) -> ("error out"=w3206:errorcluster, "file name out"=w3200:string)  [unwired: 9 in]
                    n2173 = call "FILE PATH CREATION.vi"("error in"=w3206, "FILE NAME :"=w3200) -> ("FILE OUT"=w3199:path)  [unwired: 8 in, 1 out]
                    n2174 = Concatenate Strings(w3200, ".dgf" ("Substring")) -> (w3205:string)
                    n2175 = Concatenate Strings(w3200, ".duf" ("Substring")) -> (w3201:string)
                    n2176 = Multiply(x=w3194, y=1.0) -> (x*y=w3227:dbl)
                    n2177 = Build Path(base path=w3199, name or relative path=w3205) -> (appended path=w3198:path)
                    n2178 = Build Path(base path=w3199, name or relative path=w3201) -> (appended path=w3197:path)
                    n2179 = Number To Fractional String(number=w3227, width (-)=i16 5, precision (6)=i16 2) -> (F-format string=w3235:string)  [unwired: 1 in]
                    n2180 = local read "Fuel Discription :"() -> (w3223:string)
                    n2181 = local read "Batch Ref Num :"() -> (w3211:string)
                    n2182 = Get Date/Time String(date format (0)=enum16{"short", "long", "abbreviated"}."short") -> (date string=w3246:string, time string=w3243:string)  [unwired: 2 in]
                    n2183 = local read "Remarks :"() -> (w3222:string)
                    n2184 = Concatenate Strings("Load :- " ("Substring"), w3235, " grams ," ("Substring")) -> (w3234:string)
                    n2185 = local read "String 41"() -> (w3214:string)
                    n2186 = Concatenate Strings(w3223) -> (w3224:string)
                    n2187 = Concatenate Strings(w3211) -> (w3210:string)
                    n2188 = Concatenate Strings("tested by") -> (w3218:string)
                    n2189 = Concatenate Strings("(" ("Substring"), w3246, ")" ("Substring"), w3243) -> (w3216:string)
                    "concatenated string" <- w3216
                    n2190 = Concatenate Strings(w3222, "," ("string")) -> (w3221:string)
                    n2191 = Concatenate Strings("  TIME;      COF;       STROKE;     AIR TEMP;  TEMP;  HUMIDITY;  ECR; PID-OUT; FREQUENCY" ("Substring"), "\r") -> (w3230:string)
                    n2192 = Concatenate Strings(w3214, w3213, "Fuel Discription :-" ("Substring"), w3224, w3213, w3234, w3213, "Batch Ref Num :-" ("Substring"), w3210, w3213, " Remarks :- " ("Substring"), w3221, w3213, " Date :- " ("Substring"), w3216, w3213, "Tested By :-" ("Substring"), w3218) -> (w3228:string)
                    "REMARKS" <- w3228
                    n2193 = call <vilib>:"Write Characters To File.vi"("append to file? (new file:F)"=FALSE, "character string"=w3230, "file path (dialog if empty)"=w3198) -> ()  [unwired: 2 in, 1 out]
                    n2194 = call <vilib>:"Write Characters To File.vi"("append to file? (new file:F)"=FALSE, "character string"=w3228, "file path (dialog if empty)"=w3197) -> ()  [unwired: 2 in, 1 out]
                  }
                  frame #2 {
                    n2195 = local write "Cycles elapsed"(0 ("Cycles elapsed")) -> ()
                    n2196 = local write "cyclecount"(0 ("cyclecount")) -> ()
                    n2197 = local write "Save & Continue"(FALSE ("OK")) -> ()
                    n2198 = local write "autostrtflg"(TRUE ("autostrtflg")) -> ()
                    n2199 = local write "Save"(FALSE ("Save")) -> ()
                    n2200 = Get Date/Time In Seconds() -> (seconds since 1Jan1904=w3253:timestamp)
                    n2201 = To Double Precision Float(number=w3253) -> (double precision float=w3252:dbl)
                    n2202 = local write "acq timer"(w3252) -> ()
                    n2203 = One Button Dialog(message="Please ensure sample is mounted properly and machine is ready in all aspects for testing !", button name ("OK")="Ok") -> ()  [unwired: 1 out]
                  }
                  frame #3 {
                    n2204 = stacked-sequence {
                      frame #0 {
                        n2205 = local write "Main Dashboard Buttons"(T1."Dashboard" ("Main Dashboard Buttons")) -> ()
                        n2206 = local write "Main Tab"(T2."Acquire" ("Main Tab")) -> ()
                      }
                      frame #1 {
                        n2207 = local write "EVENT LOG"("" ("EVENT LOG")) -> ()
                      }
                      frame #2 {
                        n2208 = Wait (ms)(milliseconds to wait=u32 50) -> ()  [unwired: 1 out]
                      }
                      frame #3 {
                        n2209 = disable-structure shown="Disabled" {
                          frame Disabled {
                            n2210 = local read "EVENT LOG"() -> (w3265:string)
                            n2211 = call "Event Log.vi"("Content"="Test Details", "EVENT LOG"=w3265) -> ("EVENT LOG"=w3264:string)  [unwired: 8 in, 1 out]
                            n2212 = local write "EVENT LOG"(w3264) -> ()
                          }
                          frame Enabled {
                          }
                        }
                      }
                      frame #4 {
                        n2213 = Wait (ms)(milliseconds to wait=u32 50) -> ()  [unwired: 1 out]
                      }
                      frame #5 {
                        n2214 = local read "FILE"() -> (w3267:string)
                        n2215 = Concatenate Strings("File Name :" ("Content"), w3267) -> (w3268:string)
                        n2216 = local read "EVENT LOG"() -> (w3271:string)
                        n2217 = call "Event Log.vi"("Content"=w3268, "EVENT LOG"=w3271) -> ("EVENT LOG"=w3270:string)  [unwired: 8 in, 1 out]
                        n2218 = local write "EVENT LOG"(w3270) -> ()
                      }
                      frame #6 {
                        n2219 = Wait (ms)(milliseconds to wait=u32 50) -> ()  [unwired: 1 out]
                      }
                      frame #7 {
                        n2220 = local read "Batch Ref Num :"() -> (w3273:string)
                        n2221 = Concatenate Strings("Batch Ref No :" ("Content"), w3273) -> (w3274:string)
                        n2222 = local read "EVENT LOG"() -> (w3277:string)
                        n2223 = call "Event Log.vi"("Content"=w3274, "EVENT LOG"=w3277) -> ("EVENT LOG"=w3276:string)  [unwired: 8 in, 1 out]
                        n2224 = local write "EVENT LOG"(w3276) -> ()
                      }
                      frame #8 {
                        n2225 = Wait (ms)(milliseconds to wait=u32 50) -> ()  [unwired: 1 out]
                      }
                      frame #9 {
                        n2226 = local read "tested by"() -> (w3279:string)
                        n2227 = Concatenate Strings("Tested By :" ("Content"), w3279) -> (w3280:string)
                        n2228 = local read "EVENT LOG"() -> (w3283:string)
                        n2229 = call "Event Log.vi"("Content"=w3280, "EVENT LOG"=w3283) -> ("EVENT LOG"=w3282:string)  [unwired: 8 in, 1 out]
                        n2230 = local write "EVENT LOG"(w3282) -> ()
                      }
                      frame #10 {
                        n2231 = Wait (ms)(milliseconds to wait=u32 50) -> ()  [unwired: 1 out]
                      }
                      frame #11 {
                        n2232 = local read "TEST STANDARD"() -> (w3286:T3)
                        n2233 = case shown="\"ASTM D6079\", Default" w3286 {
                          tunnel: ["ASTM D6079" "ISO 12156" "CEC F-096-A-06" "Custom"] -> w3285
                          frame "ASTM D6079", Default {
                          }
                          frame "ISO 12156" {
                          }
                          frame "CEC F-096-A-06" {
                          }
                          frame "Custom" {
                          }
                        }
                        n2234 = Concatenate Strings("Test Standard :" ("Content"), w3285) -> (w3287:string)
                        n2235 = local read "EVENT LOG"() -> (w3290:string)
                        n2236 = call "Event Log.vi"("Content"=w3287, "EVENT LOG"=w3290) -> ("EVENT LOG"=w3289:string)  [unwired: 8 in, 1 out]
                        n2237 = local write "EVENT LOG"(w3289) -> ()
                      }
                      frame #12 {
                        n2238 = Wait (ms)(milliseconds to wait=u32 50) -> ()  [unwired: 1 out]
                      }
                      frame #13 {
                        n2239 = local read "Fuel Discription :"() -> (w3296:string)
                        n2240 = Concatenate Strings("Fuel Description :" ("Content"), w3296) -> (w3297:string)
                        n2241 = local read "EVENT LOG"() -> (w3300:string)
                        n2242 = call "Event Log.vi"("Content"=w3297, "EVENT LOG"=w3300) -> ("EVENT LOG"=w3299:string)  [unwired: 8 in, 1 out]
                        n2243 = local write "EVENT LOG"(w3299) -> ()
                      }
                      frame #14 {
                        n2244 = Wait (ms)(milliseconds to wait=u32 50) -> ()  [unwired: 1 out]
                      }
                      frame #15 {
                        n2245 = local read "Remarks :"() -> (w3302:string)
                        n2246 = Concatenate Strings("Remarks :" ("Content"), w3302) -> (w3303:string)
                        n2247 = local read "EVENT LOG"() -> (w3306:string)
                        n2248 = call "Event Log.vi"("Content"=w3303, "EVENT LOG"=w3306) -> ("EVENT LOG"=w3305:string)  [unwired: 8 in, 1 out]
                        n2249 = local write "EVENT LOG"(w3305) -> ()
                      }
                      frame #16 {
                        n2250 = Wait (ms)(milliseconds to wait=u32 50) -> ()  [unwired: 1 out]
                      }
                      frame #17 {
                        n2251 = local read "Operator ID"() -> (w3308:string)
                        n2252 = Concatenate Strings("Operator ID :" ("Content"), w3308) -> (w3310:string)
                        n2253 = local read "EVENT LOG"() -> (w3312:string)
                        n2254 = call "Event Log.vi"("Content"=w3310, "EVENT LOG"=w3312) -> ("EVENT LOG"=w3311:string)  [unwired: 8 in, 1 out]
                        n2255 = local write "EVENT LOG"(w3311) -> ()
                      }
                      frame #18 {
                        n2256 = Wait (ms)(milliseconds to wait=u32 50) -> ()  [unwired: 1 out]
                      }
                      frame #19 {
                        n2257 = disable-structure shown="Disabled" {
                          frame Disabled {
                            n2258 = local read "EVENT LOG"() -> (w3316:string)
                            n2259 = call "Event Log.vi"("Content"="Test Parameter", "EVENT LOG"=w3316) -> ("EVENT LOG"=w3315:string)  [unwired: 8 in, 1 out]
                            n2260 = local write "EVENT LOG"(w3315) -> ()
                          }
                          frame Enabled {
                          }
                        }
                      }
                      frame #20 {
                        n2261 = Wait (ms)(milliseconds to wait=u32 50) -> ()  [unwired: 1 out]
                      }
                      frame #21 {
                        n2262 = local read "Set Hz"() -> (w3320:dbl)
                        n2263 = Number To Fractional String(number=w3320, precision (6)=i16 2) -> (F-format string=w3319:string)  [unwired: 2 in]
                        n2264 = Concatenate Strings("Set Frequency [Hz] :" ("Content"), w3319) -> (w3322:string)
                        n2265 = local read "EVENT LOG"() -> (w3324:string)
                        n2266 = call "Event Log.vi"("Content"=w3322, "EVENT LOG"=w3324) -> ("EVENT LOG"=w3323:string)  [unwired: 8 in, 1 out]
                        n2267 = local write "EVENT LOG"(w3323) -> ()
                      }
                      frame #22 {
                        n2268 = Wait (ms)(milliseconds to wait=u32 50) -> ()  [unwired: 1 out]
                      }
                      frame #23 {
                        n2269 = local read "NORMAL LOAD"() -> (w3327:dbl)
                        n2270 = Number To Fractional String(number=w3327, precision (6)=i16 2) -> (F-format string=w3328:string)  [unwired: 2 in]
                        n2271 = Concatenate Strings("Applied Load [grams] :" ("Content"), w3328) -> (w3330:string)
                        n2272 = local read "EVENT LOG"() -> (w3332:string)
                        n2273 = call "Event Log.vi"("Content"=w3330, "EVENT LOG"=w3332) -> ("EVENT LOG"=w3331:string)  [unwired: 8 in, 1 out]
                        n2274 = local write "EVENT LOG"(w3331) -> ()
                      }
                      frame #24 {
                        n2275 = Wait (ms)(milliseconds to wait=u32 50) -> ()  [unwired: 1 out]
                      }
                      frame #25 {
                        n2276 = local read "Set Strk"() -> (w3335:dbl)
                        n2277 = Number To Fractional String(number=w3335, precision (6)=i16 2) -> (F-format string=w3336:string)  [unwired: 2 in]
                        n2278 = Concatenate Strings("Set Stroke [mm] :" ("Content"), w3336) -> (w3338:string)
                        n2279 = local read "EVENT LOG"() -> (w3340:string)
                        n2280 = call "Event Log.vi"("Content"=w3338, "EVENT LOG"=w3340) -> ("EVENT LOG"=w3339:string)  [unwired: 8 in, 1 out]
